vi "Init.vi"(8 "error in":errorcluster, 9 "Values":refnum<class "Value.lvclass">[](array[class]), 10 "Keys":refnum<class "Key Name.lvclass">[](array[class]), 11 "VAR in":refnum<class "VAR.lvclass">) -> (0 "error out":errorcluster, 3 "VAR out":refnum<class "VAR.lvclass">)   [LabVIEW 2024, in "Electronic Datasheet.lvlib" / "VAR.lvclass"]
uses:
  VAR.lvclass
  Keyname/Key Name.lvclass
  Value/Value.lvclass
  Object Type/Object Type Base.lvclass
  VAR.lvclass/VAR.ctl
  Electronic Datasheet.lvlib
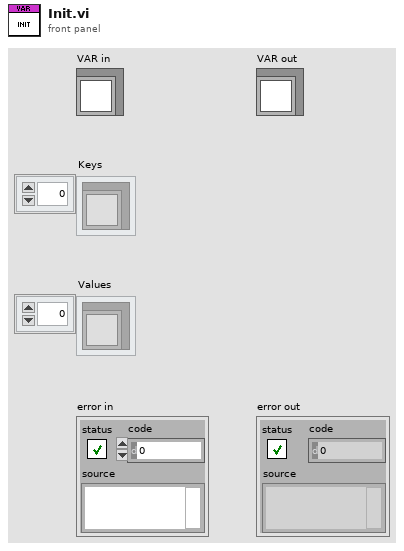
[diagram p1: front panel]
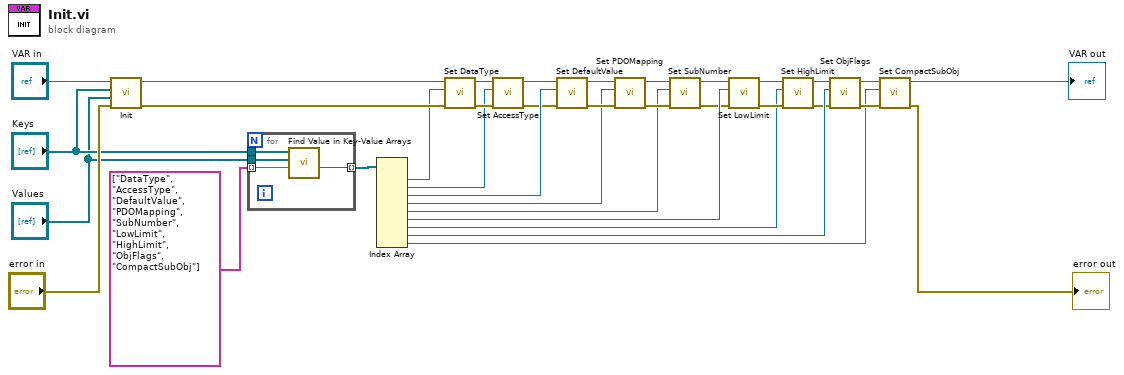
[diagram p0: block diagram]
diagram:
  n1 = call-parent "Init.vi"("error in"="error in", "Values"="Values", "Keys"="Keys", "Object Type in"="VAR in") -> ("error out"=w32:errorcluster, "Object Type out"=w33:refnum<class "VAR.lvclass">)  [unwired: 6 in]
  n2 = for {
    tunnel: "Keys" -> [w39]
    tunnel: "Values" -> [w38]
    tunnel: [w37] -> w28 mode=indexing
    tunnel: string[] ["DataType", "AccessType", "DefaultValue", "PDOMapping", "SubNumber", "LowLimit", "HighLimit", "ObjFlags", "CompactSubObj"] -> [w36] mode=indexing
    n3 = call "Find Value in Key-Value Arrays.vi"("Key Name"=w36, "Values"=w38, "Keys"=w39) -> ("Value"=w37:refnum<class "Value.lvclass">)  [unwired: 5 in, 3 out]
  }
  n4 = Index Array(array=w28) -> (element #1=w27:refnum<class "Value.lvclass">, element #2=w24:refnum<class "Value.lvclass">, element #3=w23:refnum<class "Value.lvclass">, element #4=w18:refnum<class "Value.lvclass">, element #5=w15:refnum<class "Value.lvclass">, element #6=w13:refnum<class "Value.lvclass">, element #7=w10:refnum<class "Value.lvclass">, element #8=w8:refnum<class "Value.lvclass">, element #9=w4:refnum<class "Value.lvclass">)  [unwired: 9 in]
  n5 = call-dynamic "Set DataType.vi"("error in"=w32, "Value"=w27, "Object Type in"=w33) -> ("error out"=w25:errorcluster, "Object Type out"=w29:refnum<class "VAR.lvclass">)  [unwired: 7 in]
  n6 = call-dynamic "Set AccessType.vi"("error in"=w25, "Value"=w24, "Object Type in"=w29) -> ("error out"=w22:errorcluster, "Object Type out"=w26:refnum<class "VAR.lvclass">)  [unwired: 7 in]
  n7 = call-dynamic "Set DefaultValue.vi"("error in"=w22, "Value"=w23, "Object Type in"=w26) -> ("error out"=w19:errorcluster, "Object Type out"=w21:refnum<class "VAR.lvclass">)  [unwired: 7 in]
  n8 = call-dynamic "Set PDOMapping.vi"("error in"=w19, "Value"=w18, "Object Type in"=w21) -> ("error out"=w16:errorcluster, "Object Type out"=w20:refnum<class "VAR.lvclass">)  [unwired: 7 in]
  n9 = call-dynamic "Set SubNumber.vi"("error in"=w16, "Value"=w15, "Object Type in"=w20) -> ("error out"=w1:errorcluster, "Object Type out"=w17:refnum<class "VAR.lvclass">)  [unwired: 7 in]
  n10 = call-dynamic "Set LowLimit.vi"("error in"=w1, "Value.lvclass"=w13, "Object Type in"=w17) -> ("error out"=w11:errorcluster, "Object Type out"=w14:refnum<class "VAR.lvclass">)  [unwired: 7 in]
  n11 = call-dynamic "Set HighLimit.vi"("error in"=w11, "Value"=w10, "Object Type in"=w14) -> ("error out"=w2:errorcluster, "Object Type out"=w12:refnum<class "VAR.lvclass">)  [unwired: 7 in]
  n12 = call-dynamic "Set ObjFlags.vi"("error in"=w2, "Value"=w8, "Object Type in"=w12) -> ("error out"=w5:errorcluster, "Object Type out"=w9:refnum<class "VAR.lvclass">)  [unwired: 7 in]
  n13 = call-dynamic "Set CompactSubObj.vi"("error in"=w5, "Value"=w4, "Object Type in"=w9) -> ("error out"=→"error out":errorcluster, "Object Type out"=→"VAR out":refnum<class "VAR.lvclass">)  [unwired: 7 in]
